vi "Different Error.vi"() -> ()   [LabVIEW 2017, in "Transparent Assertions.Tests.lvlib" / "Assert Error Code.lvlib"]
uses:
  Assert Error Code.lvlib
  <vilib>/Utility/error.llb/Error Cluster From Error Code.vi
  <vilib>/ErrorRing/Error Ring.xnode
  src/Transparent Assertions/Transparent Assertions.lvlib
panel:
  out "error out":errorcluster
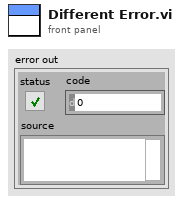
[diagram p1: front panel]
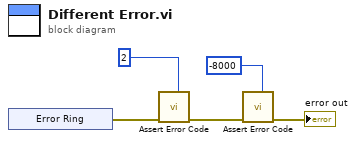
[diagram p0: block diagram]
diagram:
  n1 = xnode "Error Ring"() -> ("error out"=w3:errorcluster)
  n2 = call "Assert Error Code.vi"("Expected"=2, "error in (no error)"=w3) -> ("error out"=w5:errorcluster)  [unwired: 9 in]
  n3 = call "Assert Error Code.vi"("Expected"=-8000, "error in (no error)"=w5) -> ("error out"=→"error out":errorcluster)  [unwired: 9 in]
